vi "FreeCOM.vi"() -> ()   [LabVIEW 2014]
uses:
  <vilib>/Platform/TimedLoop/XDataNode/timing_clust.ctl
  <vilib>/Platform/TimedLoop/XDataNode/nitl_modes.ctl
  <vilib>/Platform/TimedLoop/XDataNode/wakeup.ctl
  <vilib>/Instr/_visa.llb/VISA Configure Serial Port (Instr).vi
  <vilib>/Utility/file.llb/Write To Spreadsheet File (string).vi
  <vilib>/Utility/file.llb/Write To Spreadsheet File (I64).vi
  <vilib>/Utility/file.llb/Read From Spreadsheet File (I64).vi
  <vilib>/Platform/TimedLoop/XDataNode/XDataNode.xnode
  <vilib>/Platform/TimedLoop/XDataNode/XDNodeRunTimeDep.lvlib
  <vilib>/Analysis/NI_AALBase.lvlib
  <vilib>/httpClient/LabVIEWHTTPClient.lvlib
  <vilib>/httpClient/POSTBuffer.vi
panel:
  out "字符串 2":string
  out "串口状态":bool
  out "百度纬度":dbl=50.0 format="%.10f"
  out "百度经度":dbl=50.0 format="%.10f"
  out "滤波后的历史数据":i16[][](array[numeric])
  out "04最新":i16[](array[numeric])
  out "基准时间":dbl format="%#_13g"
  out "存读的历史数据":i16[][](array[numeric])
  out "F2最新":i16[](array[numeric])
  out "F1最新":i16[](array[numeric])
  out "02最新":i16[](array[numeric])
  in  "选项卡控件":enum32{"采集界面", "地图", "设置"}(tab)
  out "波形图":i16[][](graph)
  in  "端口号":u16(ring) items=["COM1", "COM2", "COM3", "COM4", "COM5", "COM6", "COM7", "COM8", "COM9", "COM10"]
  in  "计时开关":bool
  in  "读取按钮":bool
  in  "保存按钮":bool
  out "转速":dbl(knob) scale=0.0..100.0
  out "轮速0":dbl(knob) scale=0.0..10.0
  out "档位":dbl format="%#_3g"
  out "水温":dbl(slide) scale=20.0..120.0
  out "电池电压":dbl(slide) scale=0.0..20.0
  out "节流阀位置":dbl(slide) scale=0.0..100.0
  out "前向加速度":dbl
  out "侧向加速度":dbl
  out "纵向加速度":dbl
  out "前向角速度":dbl
  out "侧向角速度":dbl
  out "纵向角速度":dbl
  out "误码":bool
  in  "open":bool
  in  "VISA资源名称":refnum<visa-resource-name>
  in  "波特率":u16(ring) caption="Baud" items=["115200", "9600"]
  out "时间差":dbl format="%#.3g秒"
  in  "侧向G值":cluster{dbl, dbl}(slide) caption="AccX图显" scale=-2.0..2.0
  in  "清除数据":bool
  in  "地图缩放":u8(slide) scale=1.0..19.0
  out "定位模式":string
  out "定位状态":dbl
  out "海拔":dbl
  in  "WebBrowser":refnum<k7>(container) caption="网页浏览器"
  out "纬度":dbl format="%#.10f"
  out "经度":dbl format="%#.10f"
  out "卫星数量":dbl
  out "地速":dbl
  out "航向":dbl
  out "航向图":picture caption="航向"
  in  "显示游标":bool
  in  "G值校准常量":dbl
  in  "串口模拟开关":bool
  out "FA数据接收（字符消息）":string caption="接收区"
  in  "发送区":string
  in  "send":bool
  in  "换行":bool
  out "TX":dbl
  out "RX":dbl
  in  "滤波系数调整":i16(slide) scale=0.0..5.0
  out "计数器":dbl
  out "历史数据05":i16[][](array[numeric])
  out "历史数据F2":i16[][](array[numeric])
  out "历史数据F1":i16[][](array[numeric])
  out "历史数据04":i16[][](array[numeric])
  out "历史数据03":i16[][](array[numeric])
  out "历史数据02":i16[][](array[numeric])
  out "历史数据01":i16[][](array[numeric])
  out "提取缓存":i64[](array[numeric])
  # "用户使用"
  # "Count"
  # "开发人员使用"
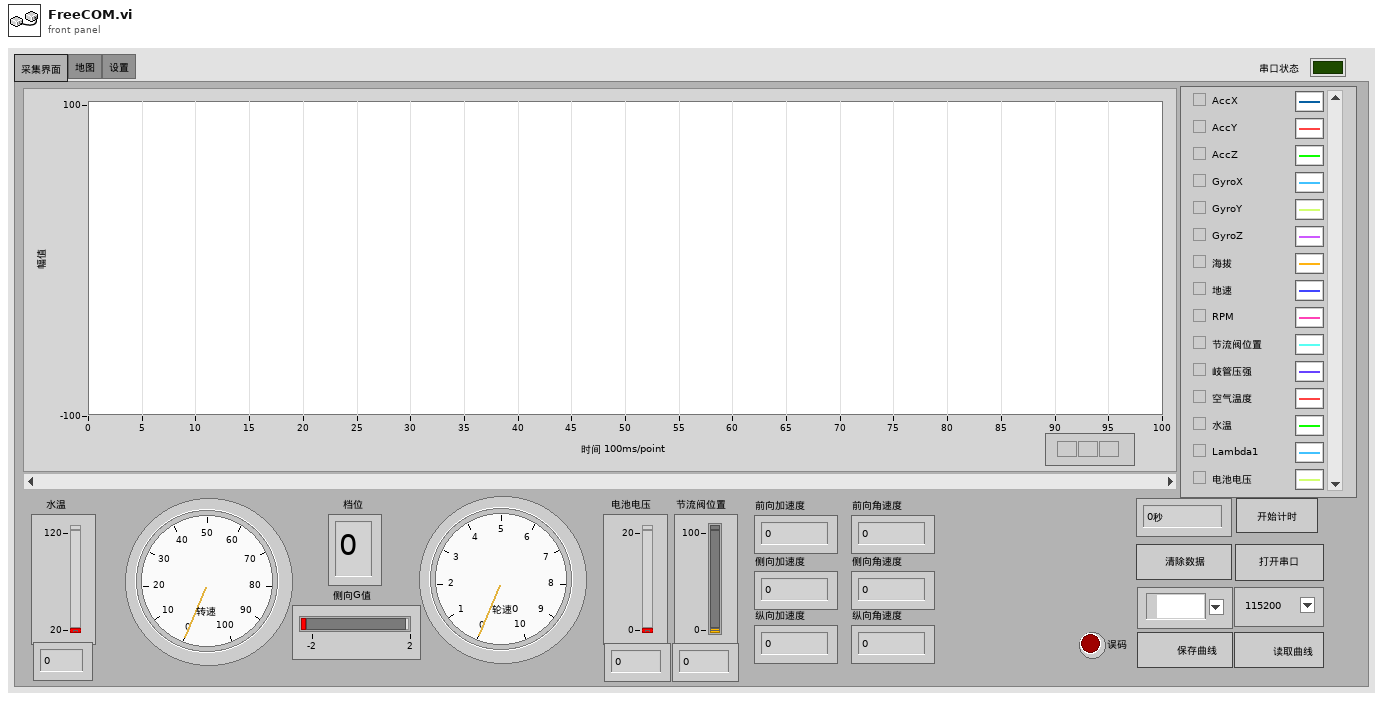
[diagram p1: front panel]
types:
  T1 = typedef "XDNodeRunTimeDep.lvlib/timing_clust.ctl" = cluster{"Expected End [f-1]":u64, "Actual End [f-1]":u64, "Finished Late? [f-1]":bool, "Expected End [i-1]":u64, "Actual End [i-1]":u64, "Finished Late? [i-1]":bool, "Expected Start [i]":u64, "Actual Start [i]":u64, "Expected Start [f]":u64, "Actual Start [f]":u64, "Source Name":string, "Structure Name":string, "Period":i64, "Deadline":i64, "Offset":i64, "Start":i64, "Priority":i32, "Timeout":i32, "Mode":T2, "Wakeup Reason":T3, "Error":errorcluster, "Source Type":string, "Secondary Source Type":string, "Global End Time":u64, "Global Start Time":u64, "Frame Duration":u64, "Iteration Duration":u64, "Assigned CPU":i32, "I/O Scan Engine Mode":u32}
  T2 = typedef "XDNodeRunTimeDep.lvlib/nitl_modes.ctl" = enum32{"No Change", "Process missed periods, maintain original phase", "Discard missed periods, maintain original phase", "Process missed periods, ignore original phase", "Discard missed periods, ignore original phase"}
  T3 = typedef "XDNodeRunTimeDep.lvlib/wakeup.ctl" = enum32{"Normal", "Aborted", "Asynchronous wakeup", "Timing source error", "Timed loop error", "Timeout"}
  T4 = cluster{"maximum":dbl, "minimum":dbl, "clip to min":bool, "log?(F)":bool, "grid color":u32, "plot color":u32, "format and precision":cluster{"format":enum8{"Decimal", "Scientific", "Engineering", "Binary", "Octal", "Hex"}, "precision":u8}, "visible section":u16}
  T5 = typedef "LabVIEWHTTPClient.lvlib/ClientHandle.ctl" = refnum<k1>
  T6 = typedef "LVBoundsTypeDef.ctl" = cluster{"Width":u32, "Height":u32}
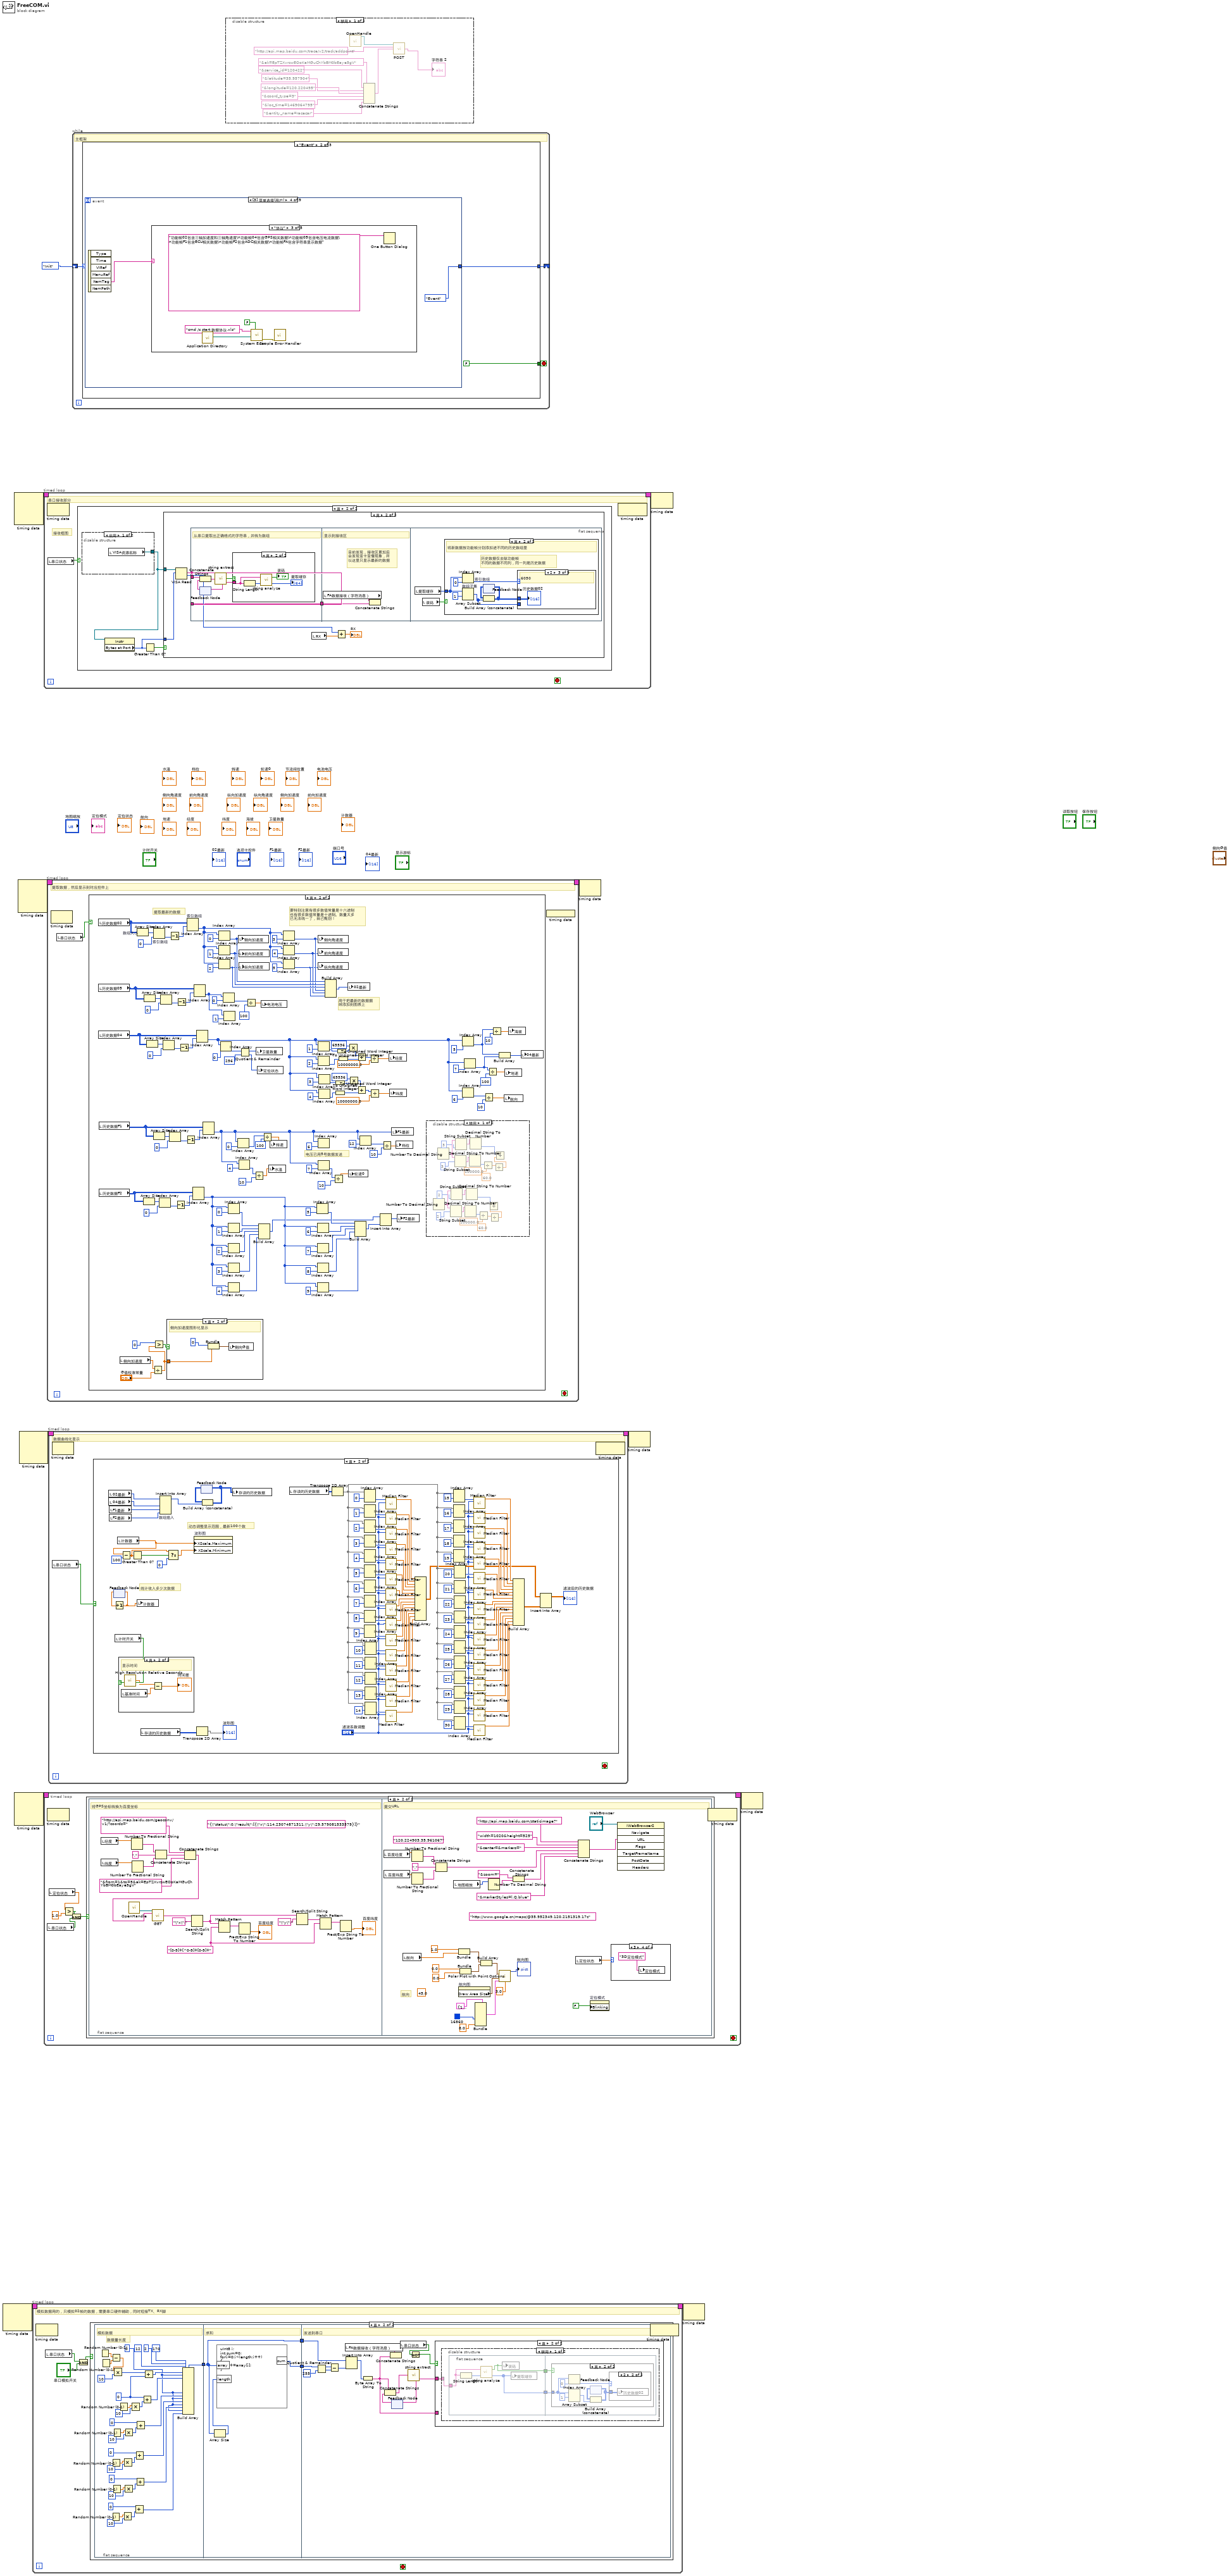
[diagram p0: block diagram]
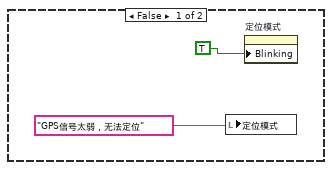
[diagram p3: hidden frame]
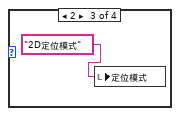
[diagram p6: hidden frame]
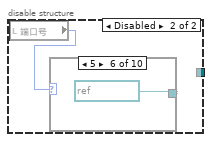
[diagram p10: hidden frame]
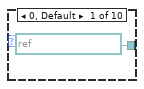
[diagram p11: hidden frame]
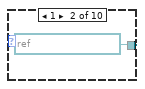
[diagram p12: hidden frame]
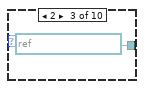
[diagram p13: hidden frame]
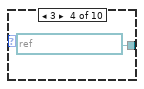
[diagram p14: hidden frame]
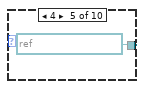
[diagram p15: hidden frame]
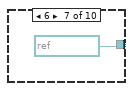
[diagram p16: hidden frame]
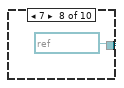
[diagram p17: hidden frame]
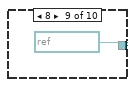
[diagram p18: hidden frame]
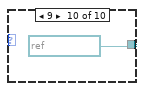
[diagram p19: hidden frame]
diagram:
  n1 = node-c288() -> (w8:T1)  [unwired: 3 in]
  n2 = node-c288() -> (w6:T1)  [unwired: 4 in]
  n3 = node-c288() -> (w2:T1)  [unwired: 4 in]
  n4 = node-c288() -> (w10:T1)  [unwired: 4 in]
  n5 = node-c288() -> (w4:T1)  [unwired: 4 in]
  n6 = timed-loop "定时循环" {
    timing: w8 -> [_]
    timing-out: [_] -> w7
    stop <- _ stop-if-true
    # "模拟数据用的，只模拟02帧的数据，需要串口硬件辅助，同时短接TX、RX脚"
    n7 = node-c288() -> ()  [unwired: 1 in, 1 out]
    n8 = local read "串口状态"() -> (w13:bool)
    n9 = And(x=w13, y="串口模拟开关") -> (x .and. y?=w12:bool)
    n10 = case shown="真" w12 {
      frame False {
      }
      frame True {
        n11 = flat-sequence "平铺式顺序结构" {
          tunnel: [w54] -> w19
          tunnel: w19 -> [w58]
          tunnel: [w57] -> w18
          tunnel: [w58] -> w17
          tunnel: w18 -> [w72]
          tunnel: w17 -> [w73]
          frame #0 {
            w46 = 0
            w24 = 0
            w55 = 170
            # "数据量长度"
            # "模拟数据"
            n12 = Random Number (0-1)() -> (number: 0 to 1=w22:dbl)
            n13 = Random Number (0-1)() -> (number: 0 to 1=w21:dbl)
            n14 = Random Number (0-1)() -> (number: 0 to 1=w28:dbl)
            n15 = Subtract(x=w22, y=w21) -> (x-y=w20:dbl)
            n16 = Random Number (0-1)() -> (number: 0 to 1=w38:dbl)
            n17 = Random Number (0-1)() -> (number: 0 to 1=w34:dbl)
            n18 = Random Number (0-1)() -> (number: 0 to 1=w43:dbl)
            n19 = Multiply ("乘")(x=w20, y=10) -> (x*y=w44:i16)
            n20 = Random Number (0-1)() -> (number: 0 to 1=w53:dbl)
            n21 = Multiply ("乘")(x=w28, y=10) -> (x*y=w26:u16)
            n22 = Multiply ("乘")(x=w38, y=10) -> (x*y=w36:u16)
            n23 = Multiply ("乘")(x=w34, y=10) -> (x*y=w32:u16)
            n24 = Multiply ("乘")(x=w43, y=10) -> (x*y=w41:u16)
            n25 = Multiply ("乘")(x=w53, y=10) -> (x*y=w51:u16)
            n26 = Add(x=0, y=w26) -> (x+y=w23:i32)
            n27 = Add(x=0, y=w36) -> (x+y=w30:i32)
            n28 = Add(x=0, y=w32) -> (x+y=w29:i32)
            n29 = Add(x=0, y=w41) -> (x+y=w39:i32)
            n30 = Add(x=w46, y=w51) -> (x+y=w50:i32)
            n31 = Add(x=w44, y=w46) -> (x+y=w45:i32)
            n32 = Build Array(w55, w55, 2, 12, w24, w45, w24, w50, w24, w39, w24, w30, w24, w29, w24, w23) -> (w54:i32[])
          }
          frame #1 {
            # "求和"
            n33 = Array Size(array=w58) -> (size(s)=w56:i32)
            n34 = formula code="uInt8 i;\nint sum=0;\nfor(i=0;i<length;i++)\n{\n sum+=array[i];\n}"("array"=w58, "length"=w56) -> ("sum"=w57:i32)
          }
          frame #2 {
            # "发送到串口"
            n35 = Quotient & Remainder(x=w72, y=255) -> (x-y*floor(x/y)=w70:i32, floor(x/y)=w69:i32)
            n36 = Subtract(x=w70, y=w69) -> (x-y=w68:i32)
            n37 = local read "FA数据接收（字符消息）"() -> (w63:string)
            n38 = Insert Into Array(array=w73, new element=w68) -> (w67:i32[])  [unwired: 1 in]
            n39 = Byte Array To String(unsigned byte array=w67) -> (string=w61:string)
            n40 = Concatenate Strings(w63, w61) -> ()  [unwired: 1 out]
            n41 = feedback #1() -> (w64:string)  [unwired: 1 in]
            n42 = Concatenate Strings(w61, w64) -> (w66:string)
            n43 = local read "串口状态"() -> (w60:bool)
            n44 = call "string extract.vi"("输入的串"=w66) -> ("输出的串"=w62:string, "剩余的串"=w65:string)  [unwired: 3 out]
            n45 = feedback-in #1(w65) -> ()
            n46 = Not(x=w60) -> (.not. x?=w59:bool)
            n47 = case shown="真" w59 {
              tunnel: w62 -> [_ w88]
              tunnel: w61 -> [w75 _]
              frame False {
                n48 = disable-structure shown="启用" {
                  disable-tunnel: [w76 _] -> w74
                  frame Enabled {
                    n49 = local read "VISA资源名称"() -> (w76:refnum<visa-resource-name>)
                  }
                  frame Disabled {
                    n50 = local read "端口号"() -> (w77:u16)
                    n51 = case shown="5" w77 {
                      tunnel: [refnum<visa-resource-name> "ASRL1::INSTR" ("VISA resource name") refnum<visa-resource-name> "ASRL2::INSTR" ("VISA resource name") refnum<visa-resource-name> "ASRL3::INSTR" ("VISA resource name") refnum<visa-resource-name> "ASRL4::INSTR" ("VISA resource name") refnum<visa-resource-name> "ASRL5::INSTR" ("VISA resource name") refnum<visa-resource-name> "COM6" ("VISA resource name") refnum<visa-resource-name> "COM7" ("VISA resource name") refnum<visa-resource-name> "COM8" ("VISA resource name") refnum<visa-resource-name> "COM9" ("VISA resource name") refnum<visa-resource-name> "COM10" ("VISA resource name")] -> _
                      frame 0, Default {
                      }
                      frame 1 {
                      }
                      frame 2 {
                      }
                      frame 3 {
                      }
                      frame 4 {
                      }
                      frame 5 {
                      }
                      frame 6 {
                      }
                      frame 7 {
                      }
                      frame 8 {
                      }
                      frame 9 {
                      }
                    }
                  }
                }
                n52 = VISA Write(VISA resource name=w74, write buffer=w75) -> ()  [unwired: 1 in, 3 out]
              }
              frame True {
                n53 = disable-structure shown="禁用" {
                  disable-tunnel: w88 -> [w89 _]
                  frame Disabled {
                    n54 = flat-sequence {
                      tunnel: w89 -> [w94]
                      tunnel: [w93] -> w91
                      tunnel: [w92] -> w90
                      tunnel: w91 -> [w97]
                      tunnel: w90 -> [w96]
                      frame #0 {
                        n55 = String Length(string=w94) -> (length=w95:i32)
                        n56 = call "string analyze.vi"("串的长度"=w95, "输入的串"=w94) -> ("输出的数组"=w92:i64[], "串正确"=w93:bool)
                        n57 = local write "误码"(w93) -> ()
                        n58 = local write "提取缓存"(w92) -> ()
                      }
                      frame #1 {
                        n59 = case shown="真" w97 {
                          tunnel: w96 -> [_ w100]
                          frame False {
                          }
                          frame True {
                            n60 = Index Array(array=w100, index=0) -> (element=w99:i64)
                            n61 = Array Subset(array=w100, index=1) -> (w104:i64[])  [unwired: 1 in]
                            n62 = feedback #2() -> (w101:i64[][])  [unwired: 1 in]
                            n63 = Build Array (concatenate)(w101, w104) -> (w98:i64[][])
                            n64 = feedback-in #2(w98) -> ()
                            n65 = case shown="2" w99 {
                              tunnel: w98 -> [_ w105]
                              frame 0, Default {
                              }
                              frame 2 {
                                n66 = local write "历史数据02"(w105) -> ()
                              }
                            }
                          }
                        }
                      }
                    }
                  }
                  frame Enabled {
                  }
                }
              }
            }
          }
        }
      }
    }
    n67 = node-c288() -> ()  [unwired: 1 in, 1 out]
  }
  n68 = timed-loop "定时循环" {
    timing: w6 -> [_]
    timing-out: [_] -> w5
    stop <- _ stop-if-true
    # "接收框图"
    # "串口接收部分"
    n69 = node-c288() -> ()  [unwired: 1 in, 1 out]
    n70 = local read "串口状态"() -> (w106:bool)
    n71 = case shown="真" w106 {
      frame False {
      }
      frame True {
        n72 = disable-structure shown="启用" {
          disable-tunnel: [w112 _] -> w109
          frame Enabled {
            n73 = local read "VISA资源名称"() -> (w112:refnum<visa-resource-name>)
          }
          frame Disabled {
            n74 = local read "端口号"() -> (w113:u16)
            n75 = case shown="5" w113 {
              tunnel: [refnum<visa-resource-name> "ASRL1::INSTR" ("VISA resource name") refnum<visa-resource-name> "ASRL2::INSTR" ("VISA resource name") refnum<visa-resource-name> "ASRL3::INSTR" ("VISA resource name") refnum<visa-resource-name> "ASRL4::INSTR" ("VISA resource name") refnum<visa-resource-name> "ASRL5::INSTR" ("VISA resource name") refnum<visa-resource-name> "COM6" ("VISA resource name") refnum<visa-resource-name> "COM7" ("VISA resource name") refnum<visa-resource-name> "COM8" ("VISA resource name") refnum<visa-resource-name> "COM9" ("VISA resource name") refnum<visa-resource-name> "COM10" ("VISA resource name")] -> _
              frame 0, Default {
              }
              frame 1 {
              }
              frame 2 {
              }
              frame 3 {
              }
              frame 4 {
              }
              frame 5 {
              }
              frame 6 {
              }
              frame 7 {
              }
              frame 8 {
              }
              frame 9 {
              }
            }
          }
        }
        n76 = property class="Instr"(reference=w109) -> ("Bytes at Port"=w111:u32)  [unwired: 1 in, 2 out]
        n77 = Greater Than 0?(x=w111) -> (x > 0?=w110:bool)
        n78 = case shown="真" w110 {
          tunnel: w109 -> [_ w130]
          tunnel: w111 -> [_ w127]
          frame False {
          }
          frame True {
            n79 = VISA Read(VISA resource name=w130, byte count=w127) -> (read buffer=w125:string, return count=w124:u32)  [unwired: 1 in, 2 out]
            n80 = flat-sequence "平铺式顺序结构" {
              tunnel: w125 -> [w132]
              tunnel: w125 -> [w131]
              tunnel: [w131] -> w126
              tunnel: w126 -> [w143]
              frame #0 {
                # "从串口提取出正确格式的字符串，并转为数组"
                n81 = feedback #3() -> (w133:string)  [unwired: 1 in]
                n82 = Concatenate Strings(w132, w133) -> (w134:string)
                n83 = call "string extract.vi"("输入的串"=w134) -> ("输出的串"=w137:string, "剩余的串"=w135:string, "输出的串非空"=w136:bool)  [unwired: 2 out]
                n84 = feedback-in #3(w135) -> ()
                n85 = case shown="真" w136 {
                  tunnel: w137 -> [_ w139]
                  frame False {
                    n86 = local write "误码"(FALSE) -> ()
                  }
                  frame True {
                    n87 = String Length(string=w139) -> (length=w142:i32)
                    n88 = call "string analyze.vi"("串的长度"=w142, "输入的串"=w139) -> ("输出的数组"=→"提取缓存":i64[], "串正确"=→"误码":bool)
                  }
                }
              }
              frame #1 {
                # "目前发现，接收区累加后\n会发现变卡变慢现象，所\n以这里只显示最新的数据"
                # "显示到接收区"
                n89 = local read "FA数据接收（字符消息）"() -> (w144:string)
                n90 = Concatenate Strings(w144, w143) -> ()  [unwired: 1 out]
              }
              frame #2 {
                n91 = local read "提取缓存"() -> (w146:i64[])
                n92 = local read "误码"() -> (w145:bool)
                n93 = case "条件结构" shown="真" w145 {
                  tunnel: w146 -> [_ w150]
                  frame False {
                  }
                  frame True {
                    # "历史数据仅去除功能帧\n不同的数据不同列，同一列是历史数据"
                    # "将新数据按功能帧分别添加进不同的历史数组里"
                    n94 = Index Array "索引数组"(array=w150, index=0) -> (element=w149:i64)
                    n95 = Array Subset "数组子集"(array=w150, index=1) -> (w147:i64[])  [unwired: 1 in]
                    n96 = feedback #4() -> (w153:i64[][])  [unwired: 1 in]
                    n97 = Build Array (concatenate)(w153, w147) -> (w148:i64[][])
                    n98 = feedback-in #4(w148) -> ()
                    n99 = case "条件结构" shown="2" w149 {
                      tunnel: w148 -> [_ w154 w155 w156 w157 w158 w159 w160 _]
                      tunnel: w147 -> [_ _ _ _ _ _ _ _ w161]
                      frame 0, Default {
                      }
                      frame 1 {
                        # "ATT"
                        "历史数据01" <- w154
                      }
                      frame 2 {
                        # "6050"
                        "历史数据02" <- w155
                      }
                      frame 3 {
                        "历史数据03" <- w156
                      }
                      frame 4 {
                        # "GPS"
                        "历史数据04" <- w157
                      }
                      frame 5 {
                        "历史数据05" <- w158
                      }
                      frame 241 {
                        # "Motec"
                        "历史数据F1" <- w159
                      }
                      frame 242 {
                        # "ADC"
                        "历史数据F2" <- w160
                      }
                      frame 250 {
                        # "FA的数据转为字符"
                        n100 = Byte Array To String(unsigned byte array=w161) -> (string=→"FA数据接收（字符消息）":string)
                      }
                    }
                  }
                }
              }
            }
            n101 = local read "RX"() -> (w129:dbl)
            n102 = Add(x=w124, y=w129) -> (x+y=→"RX":dbl)
          }
        }
      }
    }
    n103 = node-c288() -> ()  [unwired: 1 in, 1 out]
  }
  n104 = timed-loop {
    timing: w2 -> [_]
    timing-out: [_] -> w1
    stop <- _ stop-if-true
    n105 = node-c288() -> ()  [unwired: 1 in, 1 out]
    n106 = local read "串口状态"() -> (w164:bool)
    n107 = local read "定位状态"() -> (w167:dbl)
    n108 = Greater?(x=w167, y=1.0) -> (0:w165:bool)
    n109 = And(x=w165, y=w164) -> (x .and. y?=w163:bool)
    n110 = case shown="真" w163 {
      frame False {
        n111 = local write "定位模式"("GPS信号太弱，无法定位") -> ()
        n112 = property on="定位模式" class="Str"("Blinking"=TRUE) -> ()  [unwired: 2 in, 2 out]
      }
      frame True {
        n113 = flat-sequence "平铺式顺序结构" {
          frame #0 {
            w189 = "[0-9]+[^0-9]+[0-9]+"
            (unwired) "{\"status\":0,\"result\":[{\"x\":114.23074871311,\"y\":29.579081533579}]}" ("字符串 2")
            # "将GPS坐标转换为百度坐标"
            n114 = local read "经度"() -> (w174:dbl)
            n115 = local read "纬度"() -> (w175:dbl)
            n116 = call <vilib>:"OpenHandle.vi"() -> ("client handle out"=w187:T5)  [unwired: 14 in, 1 out]
            n117 = Number To Fractional String(number=w174) -> (F-format string=w178:string)  [unwired: 3 in]
            n118 = Number To Fractional String(number=w175) -> (F-format string=w176:string)  [unwired: 3 in]
            n119 = Concatenate Strings(w178, ",", w176) -> (w172:string)
            n120 = Concatenate Strings("http://api.map.baidu.com/geoconv/v1/?coords=", w172, "&from=1&to=5&ak=EpTZXvrzwEOoKaMGuChYbBM0bEaye5gV") -> (w170:string)
            n121 = call <vilib>:"GET.vi"("client handle"=w187, "url"=w170) -> ("body"=w188:string)  [unwired: 10 in, 3 out]
            n122 = Search/Split String(string=w188, search string/char (-)="\"x\":") -> (match + rest of string=w185:string)  [unwired: 1 in, 2 out]
            n123 = Match Pattern(string=w185, regular expression=w189) -> (match substring=w186:string)  [unwired: 1 in, 3 out]
            n124 = Fract/Exp String To Number(string=w186) -> (number=→"百度经度":dbl)  [unwired: 3 in, 1 out]
            n125 = Search/Split String(string=w185, search string/char (-)="\"y\":") -> (match + rest of string=w182:string)  [unwired: 1 in, 2 out]
            n126 = Match Pattern(string=w182, regular expression=w189) -> (match substring=w184:string)  [unwired: 1 in, 3 out]
            n127 = Fract/Exp String To Number(string=w184) -> (number=→"百度纬度":dbl)  [unwired: 3 in, 1 out]
          }
          frame #1 {
            (unwired) "http://www.google.cn/maps/@35.952349,120.2151319,17z"
            (unwired) 45.0
            (unwired) "120.224903,35.961067"
            # "航向"
            # "提交URL"
            n128 = local read "百度经度"() -> (w202:dbl)
            n129 = local read "百度纬度"() -> (w201:dbl)
            n130 = local read "航向"() -> (w191:dbl)
            n131 = Number To Fractional String(number=w202) -> (F-format string=w200:string)  [unwired: 3 in]
            n132 = Number To Fractional String(number=w201) -> (F-format string=w198:string)  [unwired: 3 in]
            n133 = Concatenate Strings(w200, ",", w198) -> (w192:string)
            n134 = local read "地图缩放"() -> (w196:u8)
            n135 = Bundle(1.0, "航向"=w191) -> (w209:cluster{dbl, " 航向":dbl})  [unwired: 1 in]
            n136 = property on="航向图" class="Pict"() -> ("Draw Area Size"=w205:T6)  [unwired: 2 in, 2 out]
            n137 = Bundle(0.0, 0.0) -> (w210:cluster{dbl, dbl})  [unwired: 1 in]
            n138 = Bundle(cluster=T4 {"maximum"=1.0, "minimum"=0.0, "clip to min"=FALSE, "log?(F)"=FALSE, "grid color"=6710886, "plot color"=65280, "format and precision"={"format"=enum."Decimal", "precision"=1}, "visible section"=0} ("Polar Graph Attributes"), "plot color"=u32 16860, "visible section"=8.0) -> (w213:T4)  [unwired: 6 in]
            n139 = Build Array(w209, w210) -> (w211:cluster{dbl, " 航向":dbl}[])
            n140 = Number To Decimal String(number=w196) -> (decimal integer string=w195:string)  [unwired: 1 in]
            n141 = call <vilib>:"Polar Plot with Point Options.vi"("data array [mag, phase (deg)]"=w211, "dimensions (w,h)"=w205, "polar attributes"=w213, "Size"=3.0) -> ("new picture"=→"航向图":picture)  [unwired: 11 in]
            n142 = Concatenate Strings("&zoom=", w195) -> (w194:string)
            n143 = local read "定位状态"() -> (w203:dbl)
            n144 = Concatenate Strings("http://api.map.baidu.com/staticimage?", "width=1020&height=525", "&center=&markers=", w192, w194, "&markerStyles=l,Q,blue") -> (w190:string)
            n145 = property on="定位模式" class="Str"("Blinking"=FALSE) -> ()  [unwired: 2 in, 2 out]
            n146 = case shown="3" w203 {
              frame 0, Default {
              }
              frame 1 {
              }
              frame 2 {
                n147 = local write "定位模式"("2D定位模式") -> ()
              }
              frame 3 {
                n148 = local write "定位模式"("3D定位模式") -> ()
              }
            }
            n149 = invoke class="IWebBrowser2" method="Navigate"(reference="WebBrowser", "URL"=w190) -> ()  [unwired: 6 in, 8 out]
          }
        }
      }
    }
    n150 = node-c288() -> ()  [unwired: 1 in, 1 out]
  }
  n151 = timed-loop "定时循环" {
    timing: w10 -> [_]
    timing-out: [_] -> w9
    stop <- _ stop-if-true
    # "提取数据，然后显示到对应控件上"
    n152 = node-c288() -> ()  [unwired: 1 in, 1 out]
    n153 = local read "串口状态"() -> (w226:bool)
    n154 = case shown="真" w226 {
      frame False {
      }
      frame True {
        # "要特别注意有很多数值常量是十六进制\n也有很多数值常量是十进制。数量太多\n已无法统一了，自己甄别！"
        # "用于把最新的数据捆\n绑添加到图表上"
        # "提取最新的数据"
        # "电压已用5号数据发送"
        n155 = local read "历史数据02"() -> (w299:i16[][])
        n156 = local read "历史数据05"() -> (w357:i16[][])
        n157 = local read "历史数据04"() -> (w318:i16[][])
        n158 = local read "历史数据F1"() -> (w356:i16[][])
        n159 = local read "历史数据F2"() -> (w345:i16[][])
        n160 = local read "侧向加速度"() -> (w275:dbl)
        n161 = Array Size "数组大小"(array=w299) -> (size(s)=w298:i32[])
        n162 = Array Size(array=w345) -> (size(s)=w341:i32[])
        n163 = Array Size(array=w357) -> (size(s)=w309:i32[])
        n164 = Array Size(array=w318) -> (size(s)=w314:i32[])
        n165 = Divide(x=w275, y="G值校准常量") -> (x/y=w274:dbl)
        n166 = Index Array "索引数组"(array=w298, index=0) -> (element=w301:i32)
        n167 = Array Size(array=w356) -> (size(s)=w332:i32[])
        n168 = Greater?(x=i16 0, y=w274) -> (0:w282:bool)
        n169 = Index Array(array=w341, index=0) -> (element=w343:i32)
        n170 = Index Array(array=w309, index=0) -> (element=w311:i32)
        n171 = Index Array(array=w314, index=0) -> (element=w316:i32)
        n172 = case "条件结构" shown="真" w282 {
          tunnel: w274 -> [w381 w384]
          frame False {
            n173 = Bundle(w381, i16 0) -> (w382:cluster{dbl, i16})  [unwired: 1 in]
            n174 = local write "侧向G值"(w382) -> ()
          }
          frame True {
            # "侧向加速度图形化显示"
            n175 = Bundle(i16 0, w384) -> (w385:cluster{i16, dbl})  [unwired: 1 in]
            n176 = local write "侧向G值"(w385) -> ()
          }
        }
        n177 = Decrement(x=w301) -> (x-1=w302:i32)
        n178 = Index Array(array=w332, index=0) -> (element=w334:i32)
        n179 = Decrement(x=w343) -> (x-1=w344:i32)
        n180 = Decrement(x=w311) -> (x-1=w312:i32)
        n181 = Decrement(x=w316) -> (x-1=w317:i32)
        n182 = Decrement(x=w334) -> (x-1=w335:i32)
        n183 = Index Array "索引数组"(array=w299, index (row)=w302) -> (element=w283:i16[])  [unwired: 1 in]
        n184 = Index Array(array=w345, index (row)=w344) -> (element=w359:i16[])  [unwired: 1 in]
        n185 = Index Array(array=w357, index (row)=w312) -> (element=w297:i16[])  [unwired: 1 in]
        n186 = Index Array(array=w318, index (row)=w317) -> (element=w243:i16[])  [unwired: 1 in]
        n187 = Index Array(array=w356, index (row)=w335) -> (element=w264:i16[])  [unwired: 1 in]
        n188 = Index Array(array=w283, index=0) -> (element=w272:i16)
        n189 = Index Array(array=w283, index=1) -> (element=w271:i16)
        n190 = Index Array(array=w283, index=2) -> (element=w270:i16)
        n191 = Index Array(array=w243, index=0) -> (element=w321:i16)
        n192 = Index Array(array=w297, index=0) -> (element=w262:i16)
        n193 = Index Array(array=w297, index=1) -> ()  [unwired: 1 out]
        n194 = Index Array(array=w359, index=0) -> (element=w296:i16)
        n195 = Index Array(array=w359, index=1) -> (element=w295:i16)
        n196 = Index Array(array=w359, index=2) -> (element=w293:i16)
        n197 = Index Array(array=w359, index=3) -> (element=w294:i16)
        n198 = Index Array(array=w359, index=4) -> (element=w292:i16)
        n199 = Index Array(array=w264, index=0) -> (element=w280:i16)
        n200 = local write "侧向加速度"(w272) -> ()
        n201 = local write "前向加速度"(w271) -> ()
        n202 = local write "纵向加速度"(w270) -> ()
        n203 = Index Array(array=w264, index=4) -> (element=w259:i16)
        n204 = Quotient & Remainder(x=w321, y=256) -> (x-y*floor(x/y)=w322:i32, floor(x/y)=w241:i32)
        n205 = Divide(x=w262, y=100) -> (x/y=w260:dbl)
        n206 = Divide(x=w259, y=10) -> (x/y=w257:dbl)
        n207 = local write "卫星数量"(w322) -> ()
        n208 = local write "定位状态"(w241) -> ()
        n209 = Build Array(w296, w295, w293, w294, w292) -> (w286:i16[])
        n210 = local write "电池电压"(w260) -> ()
        n211 = Divide(x=w280, y=100) -> (x/y=w278:dbl)
        n212 = local write "水温"(w257) -> ()
        n213 = local write "转速"(w278) -> ()
        n214 = Index Array(array=w283, index=3) -> (element=w269:i16)
        n215 = Index Array(array=w283, index=4) -> (element=w268:i16)
        n216 = Index Array(array=w283, index=5) -> (element=w267:i16)
        n217 = Index Array(array=w359, index=5) -> (element=w291:i16)
        n218 = Index Array(array=w359, index=6) -> (element=w290:i16)
        n219 = Index Array(array=w359, index=7) -> (element=w289:i16)
        n220 = Index Array(array=w359, index=8) -> (element=w288:i16)
        n221 = Index Array(array=w359, index=9) -> (element=w287:i16)
        n222 = local write "侧向角速度"(w269) -> ()
        n223 = local write "前向角速度"(w268) -> ()
        n224 = local write "纵向角速度"(w267) -> ()
        n225 = Index Array(array=w243, index=1) -> (element=w232:i16)
        n226 = Index Array(array=w243, index=2) -> (element=w234:i16)
        n227 = Index Array(array=w264, index=6) -> ()  [unwired: 1 out]
        n228 = Index Array(array=w264, index=7) -> (element=w255:i16)
        n229 = Index Array(array=w243, index=3) -> (element=w230:i16)
        n230 = Index Array(array=w243, index=4) -> (element=w228:i16)
        n231 = Build Array(w272, w271, w270, w269, w268, w267) -> (w266:i16[])
        n232 = Divide(x=w255, y=10) -> (x/y=w254:dbl)
        n233 = To Unsigned Word Integer(number=w230) -> (unsigned 16bit integer=w229:u16)
        n234 = To Unsigned Word Integer(number=w228) -> (unsigned 16bit integer=w227:u16)
        n235 = To Unsigned Word Integer(number=w232) -> (unsigned 16bit integer=w231:u16)
        n236 = To Unsigned Word Integer(number=w234) -> (unsigned 16bit integer=w233:u16)
        n237 = local write "02最新"(w266) -> ()
        n238 = Multiply(x=65536, y=w231) -> (x*y=w253:i32)
        n239 = Multiply(x=65536, y=w229) -> (x*y=w329:i32)
        n240 = local write "轮速0"(w254) -> ()
        n241 = Build Array(w291, w290, w289, w288, w287) -> (w285:i16[])
        n242 = Add(x=w253, y=w233) -> (x+y=w240:i32)
        n243 = Add(x=w329, y=w227) -> (x+y=w237:i32)
        n244 = Index Array(array=w264, index=12) -> (element=w273:i16)
        n245 = Divide(x=w240, y=10000000.0) -> (x/y=w238:dbl)
        n246 = Divide(x=w237, y=10000000.0) -> (x/y=w235:dbl)
        n247 = Insert Into Array(array=w286, new element=w285) -> (w284:i16[])  [unwired: 1 in]
        n248 = Divide(x=w273, y=10) -> (x/y=w276:dbl)
        n249 = local write "经度"(w238) -> ()
        n250 = local write "纬度"(w235) -> ()
        n251 = local write "F1最新"(w264) -> ()
        n252 = local write "档位"(w276) -> ()
        n253 = local write "F2最新"(w284) -> ()
        n254 = disable-structure shown="禁用" {
          frame Disabled {
            (unwired) 60.0
            (unwired) 60.0
            n255 = Number To Decimal String() -> (decimal integer string=w365:string)  [unwired: 2 in]
            n256 = Number To Decimal String() -> (decimal integer string=w375:string)  [unwired: 2 in]
            n257 = String Subset(string=w365, offset (0)=2) -> (substring=w369:string)  [unwired: 1 in]
            n258 = String Subset(string=w365, length (rest)=2) -> (substring=w364:string)  [unwired: 1 in]
            n259 = String Subset(string=w375, offset (0)=3) -> (substring=w379:string)  [unwired: 1 in]
            n260 = String Subset(string=w375, length (rest)=3) -> (substring=w374:string)  [unwired: 1 in]
            n261 = Decimal String To Number(string=w369) -> (number=w368:i32)  [unwired: 2 in, 1 out]
            n262 = Decimal String To Number(string=w364) -> (number=w361:i32)  [unwired: 2 in, 1 out]
            n263 = Decimal String To Number(string=w379) -> (number=w378:i32)  [unwired: 2 in, 1 out]
            n264 = Decimal String To Number(string=w374) -> (number=w371:i32)  [unwired: 2 in, 1 out]
            n265 = Divide(x=w368, y=100000.0) -> (x/y=w366:dbl)
            n266 = Divide(x=w378, y=100000.0) -> (x/y=w376:dbl)
            n267 = Divide(x=w366) -> (x/y=w362:dbl)  [unwired: 1 in]
            n268 = Add(x=w361, y=w362) -> (x+y=w360:dbl)
            n269 = Divide(x=w376) -> (x/y=w372:dbl)  [unwired: 1 in]
            n270 = Add(x=w371, y=w372) -> ()  [unwired: 1 out]
          }
          frame Enabled {
          }
        }
        n271 = Index Array(array=w243, index=6) -> (element=w245:i16)
        n272 = Index Array(array=w243, index=5) -> (element=w252:i16)
        n273 = Index Array(array=w243, index=7) -> (element=w248:i16)
        n274 = Divide(x=w245, y=10) -> (x/y=w242:dbl)
        n275 = Divide(x=w248, y=100) -> (x/y=w247:dbl)
        n276 = Divide(x=w252, y=10) -> (x/y=w250:dbl)
        n277 = Build Array(w252, w248) -> (w265:i16[])
        n278 = local write "航向"(w242) -> ()
        n279 = local write "地速"(w247) -> ()
        n280 = local write "海拔"(w250) -> ()
        n281 = local write "04最新"(w265) -> ()
      }
    }
    n282 = node-c288() -> ()  [unwired: 1 out]
  }
  n283 = timed-loop "定时循环" {
    timing: w4 -> [_]
    timing-out: [_] -> w3
    stop <- _ stop-if-true
    # "数据曲线化显示"
    n284 = node-c288() -> ()  [unwired: 1 in, 1 out]
    n285 = local read "串口状态"() -> (w389:bool)
    n286 = case shown="真" w389 {
      frame False {
      }
      frame True {
        # "动态调整显示范围，最新100个数"
        # "统计收入多少次数据"
        n287 = local read "02最新"() -> (w503:i16[])
        n288 = local read "04最新"() -> (w502:i16[])
        n289 = local read "F1最新"() -> (w501:i16[])
        n290 = local read "F2最新"() -> (w500:i16[])
        n291 = feedback #5() -> (w493:dbl)  [unwired: 1 in]
        n292 = Increment(x=w493) -> (x+1=w492:dbl)
        n293 = feedback-in #5(w492) -> ()
        n294 = local read "计时开关"() -> (w491:bool)
        n295 = local read "计数器"() -> (w499:dbl)
        n296 = case "条件结构" shown="真" w491 {
          frame False {
          }
          frame True {
            # "显示时间"
            n297 = local read "基准时间"() -> (w509:dbl)
            n298 = call <vilib>:"High Resolution Relative Seconds.vi"() -> ("relative seconds"=w508:dbl)
            n299 = Subtract(x=w508, y=w509) -> (x-y=→"时间差":dbl)
          }
        }
        n300 = Subtract(x=w499, y=i16 100) -> (x-y=w494:dbl)
        n301 = Greater Than 0?(x=w494) -> (x > 0?=w497:bool)
        n302 = local write "计数器"(w492) -> ()
        n303 = local read "存读的历史数据"() -> (w490:i16[][])
        n304 = Insert Into Array "数组插入"(array=w503, new element #1=w502, new element #2=w501, new element #3=w500) -> (w505:i16[])  [unwired: 1 in]
        n305 = Select(t=w494, s=w497, f=i16 0) -> (s? t:f=w496:dbl)
        n306 = property on="波形图" class="WFGraph (严格)"("XScale.Maximum"=w499, "XScale.Minimum"=w496) -> ()  [unwired: 2 in, 2 out]
        n307 = Transpose 2D Array(2D array=w490) -> (transposed array=→"波形图":i16[][])
        n308 = feedback #6() -> (w504:i16[][])  [unwired: 1 in]
        n309 = Build Array (concatenate)(w504, w505) -> (w506:i16[][])
        n310 = feedback-in #6(w506) -> ()
        n311 = local write "存读的历史数据"(w506) -> ()
        n312 = local read "存读的历史数据"() -> (w488:i16[][])
        n313 = Transpose 2D Array(2D array=w488) -> (transposed array=w441:i16[][])
        n314 = Index Array(array=w441, index (row)=i16 0) -> (element=w456:i16[])  [unwired: 1 in]
        n315 = Index Array(array=w441, index (row)=i16 1) -> (element=w454:i16[])  [unwired: 1 in]
        n316 = Index Array(array=w441, index (row)=i16 2) -> (element=w453:i16[])  [unwired: 1 in]
        n317 = Index Array(array=w441, index (row)=i16 3) -> (element=w452:i16[])  [unwired: 1 in]
        n318 = Index Array(array=w441, index (row)=i16 4) -> (element=w451:i16[])  [unwired: 1 in]
        n319 = Index Array(array=w441, index (row)=i16 5) -> (element=w450:i16[])  [unwired: 1 in]
        n320 = Index Array(array=w441, index (row)=i16 6) -> (element=w449:i16[])  [unwired: 1 in]
        n321 = Index Array(array=w441, index (row)=i16 7) -> (element=w448:i16[])  [unwired: 1 in]
        n322 = Index Array(array=w441, index (row)=i16 8) -> (element=w447:i16[])  [unwired: 1 in]
        n323 = Index Array(array=w441, index (row)=i16 9) -> (element=w446:i16[])  [unwired: 1 in]
        n324 = Index Array(array=w441, index (row)=i16 10) -> (element=w445:i16[])  [unwired: 1 in]
        n325 = Index Array(array=w441, index (row)=i16 11) -> (element=w444:i16[])  [unwired: 1 in]
        n326 = Index Array(array=w441, index (row)=i16 12) -> (element=w443:i16[])  [unwired: 1 in]
        n327 = Index Array(array=w441, index (row)=i16 13) -> (element=w442:i16[])  [unwired: 1 in]
        n328 = Index Array(array=w441, index (row)=i16 14) -> (element=w455:i16[])  [unwired: 1 in]
        n329 = call <vilib>:"Median Filter.vi"("left rank"="滤波系数调整", "X"=w456) -> ("Filtered X"=w424:dbl[])  [unwired: 8 in, 1 out]
        n330 = call <vilib>:"Median Filter.vi"("left rank"="滤波系数调整", "X"=w454) -> ("Filtered X"=w423:dbl[])  [unwired: 8 in, 1 out]
        n331 = call <vilib>:"Median Filter.vi"("left rank"="滤波系数调整", "X"=w453) -> ("Filtered X"=w422:dbl[])  [unwired: 8 in, 1 out]
        n332 = call <vilib>:"Median Filter.vi"("left rank"="滤波系数调整", "X"=w452) -> ("Filtered X"=w421:dbl[])  [unwired: 8 in, 1 out]
        n333 = call <vilib>:"Median Filter.vi"("left rank"="滤波系数调整", "X"=w451) -> ("Filtered X"=w420:dbl[])  [unwired: 8 in, 1 out]
        n334 = call <vilib>:"Median Filter.vi"("left rank"="滤波系数调整", "X"=w450) -> ("Filtered X"=w419:dbl[])  [unwired: 8 in, 1 out]
        n335 = call <vilib>:"Median Filter.vi"("left rank"="滤波系数调整", "X"=w449) -> ("Filtered X"=w418:dbl[])  [unwired: 8 in, 1 out]
        n336 = call <vilib>:"Median Filter.vi"("left rank"="滤波系数调整", "X"=w448) -> ("Filtered X"=w417:dbl[])  [unwired: 8 in, 1 out]
        n337 = call <vilib>:"Median Filter.vi"("left rank"="滤波系数调整", "X"=w447) -> ("Filtered X"=w416:dbl[])  [unwired: 8 in, 1 out]
        n338 = call <vilib>:"Median Filter.vi"("left rank"="滤波系数调整", "X"=w446) -> ("Filtered X"=w415:dbl[])  [unwired: 8 in, 1 out]
        n339 = call <vilib>:"Median Filter.vi"("left rank"="滤波系数调整", "X"=w445) -> ("Filtered X"=w414:dbl[])  [unwired: 8 in, 1 out]
        n340 = call <vilib>:"Median Filter.vi"("left rank"="滤波系数调整", "X"=w444) -> ("Filtered X"=w413:dbl[])  [unwired: 8 in, 1 out]
        n341 = call <vilib>:"Median Filter.vi"("left rank"="滤波系数调整", "X"=w443) -> ("Filtered X"=w412:dbl[])  [unwired: 8 in, 1 out]
        n342 = call <vilib>:"Median Filter.vi"("left rank"="滤波系数调整", "X"=w442) -> ("Filtered X"=w411:dbl[])  [unwired: 8 in, 1 out]
        n343 = call <vilib>:"Median Filter.vi"("left rank"="滤波系数调整", "X"=w455) -> ("Filtered X"=w410:dbl[])  [unwired: 8 in, 1 out]
        n344 = Build Array(w424, w423, w422, w421, w420, w419, w418, w417, w416, w415, w414, w413, w412, w411, w410) -> (w393:dbl[][])
        n345 = Index Array(array=w441, index (row)=i16 15) -> (element=w440:i16[])  [unwired: 1 in]
        n346 = Index Array(array=w441, index (row)=i16 16) -> (element=w439:i16[])  [unwired: 1 in]
        n347 = Index Array(array=w441, index (row)=i16 17) -> (element=w438:i16[])  [unwired: 1 in]
        n348 = Index Array(array=w441, index (row)=i16 18) -> (element=w437:i16[])  [unwired: 1 in]
        n349 = Index Array(array=w441, index (row)=i16 19) -> (element=w436:i16[])  [unwired: 1 in]
        n350 = Index Array(array=w441, index (row)=i16 20) -> (element=w435:i16[])  [unwired: 1 in]
        n351 = Index Array(array=w441, index (row)=i16 21) -> (element=w434:i16[])  [unwired: 1 in]
        n352 = Index Array(array=w441, index (row)=i16 22) -> (element=w433:i16[])  [unwired: 1 in]
        n353 = Index Array(array=w441, index (row)=i16 23) -> (element=w432:i16[])  [unwired: 1 in]
        n354 = Index Array(array=w441, index (row)=i16 24) -> (element=w431:i16[])  [unwired: 1 in]
        n355 = Index Array(array=w441, index (row)=i16 25) -> (element=w430:i16[])  [unwired: 1 in]
        n356 = Index Array(array=w441, index (row)=i16 26) -> (element=w429:i16[])  [unwired: 1 in]
        n357 = Index Array(array=w441, index (row)=i16 27) -> (element=w428:i16[])  [unwired: 1 in]
        n358 = Index Array(array=w441, index (row)=i16 28) -> (element=w427:i16[])  [unwired: 1 in]
        n359 = Index Array(array=w441, index (row)=i16 29) -> (element=w426:i16[])  [unwired: 1 in]
        n360 = Index Array(array=w441, index (row)=i16 30) -> (element=w425:i16[])  [unwired: 1 in]
        n361 = call <vilib>:"Median Filter.vi"("left rank"="滤波系数调整", "X"=w440) -> ("Filtered X"=w409:dbl[])  [unwired: 8 in, 1 out]
        n362 = call <vilib>:"Median Filter.vi"("left rank"="滤波系数调整", "X"=w439) -> ("Filtered X"=w408:dbl[])  [unwired: 8 in, 1 out]
        n363 = call <vilib>:"Median Filter.vi"("left rank"="滤波系数调整", "X"=w438) -> ("Filtered X"=w407:dbl[])  [unwired: 8 in, 1 out]
        n364 = call <vilib>:"Median Filter.vi"("left rank"="滤波系数调整", "X"=w437) -> ("Filtered X"=w406:dbl[])  [unwired: 8 in, 1 out]
        n365 = call <vilib>:"Median Filter.vi"("left rank"="滤波系数调整", "X"=w436) -> ("Filtered X"=w405:dbl[])  [unwired: 8 in, 1 out]
        n366 = call <vilib>:"Median Filter.vi"("left rank"="滤波系数调整", "X"=w435) -> ("Filtered X"=w404:dbl[])  [unwired: 8 in, 1 out]
        n367 = call <vilib>:"Median Filter.vi"("left rank"="滤波系数调整", "X"=w434) -> ("Filtered X"=w403:dbl[])  [unwired: 8 in, 1 out]
        n368 = call <vilib>:"Median Filter.vi"("left rank"="滤波系数调整", "X"=w433) -> ("Filtered X"=w402:dbl[])  [unwired: 8 in, 1 out]
        n369 = call <vilib>:"Median Filter.vi"("left rank"="滤波系数调整", "X"=w432) -> ("Filtered X"=w401:dbl[])  [unwired: 8 in, 1 out]
        n370 = call <vilib>:"Median Filter.vi"("left rank"="滤波系数调整", "X"=w431) -> ("Filtered X"=w400:dbl[])  [unwired: 8 in, 1 out]
        n371 = call <vilib>:"Median Filter.vi"("left rank"="滤波系数调整", "X"=w430) -> ("Filtered X"=w399:dbl[])  [unwired: 8 in, 1 out]
        n372 = call <vilib>:"Median Filter.vi"("left rank"="滤波系数调整", "X"=w429) -> ("Filtered X"=w398:dbl[])  [unwired: 8 in, 1 out]
        n373 = call <vilib>:"Median Filter.vi"("left rank"="滤波系数调整", "X"=w428) -> ("Filtered X"=w397:dbl[])  [unwired: 8 in, 1 out]
        n374 = call <vilib>:"Median Filter.vi"("left rank"="滤波系数调整", "X"=w427) -> ("Filtered X"=w396:dbl[])  [unwired: 8 in, 1 out]
        n375 = call <vilib>:"Median Filter.vi"("left rank"="滤波系数调整", "X"=w426) -> ("Filtered X"=w395:dbl[])  [unwired: 8 in, 1 out]
        n376 = call <vilib>:"Median Filter.vi"("left rank"="滤波系数调整", "X"=w425) -> ("Filtered X"=w394:dbl[])  [unwired: 8 in, 1 out]
        n377 = Build Array(w409, w408, w407, w406, w405, w404, w403, w402, w401, w400, w399, w398, w397, w396, w395, w394) -> (w392:dbl[][])
        n378 = Insert Into Array(array=w393, new element=w392) -> (→"滤波后的历史数据":dbl[][])  [unwired: 2 in]
      }
    }
    n379 = node-c288() -> ()  [unwired: 1 in, 1 out]
  }
  n380 = while "While循环" {
    shift-right: [w512] -> _
    shift-left: enum16{"Init", "Event", "Exit"}."Init" -> [w513]
    stop <- w514 stop-if-true
    # "主框架"
    n381 = case shown="\"Event\"" w513 {
      tunnel: [FALSE FALSE TRUE] -> w514
      tunnel: [enum16{"Init", "Event", "Exit"}."Event" w538 enum16{"Init", "Event", "Exit"}."Exit"] -> w512
      frame "Init", Default {
        w517 = FALSE
        w520 = 0.0 ("TX")
        w528 = 0
        n382 = local read "WebBrowser"() -> (w516:refnum<k7>)
        n383 = invoke class="IWebBrowser2" method="Navigate"(reference=w516, "URL"="www.map.baidu.com") -> ()  [unwired: 6 in, 8 out]
        n384 = property on="波形图" class="WFGraph (严格)"("XScale.Maximum"=100, "XScale.Minimum"=0, "YScale.Maximum"=100, "YScale.Minimum"=-100) -> ()  [unwired: 2 in, 2 out]
        n385 = local write "FA数据接收（字符消息）"("Receive Area") -> ()
        n386 = local write "滤波系数调整"(3) -> ()
        n387 = local write "G值校准常量"(16600.0 ("RX")) -> ()
        n388 = local write "误码"(FALSE) -> ()
        n389 = local write "串口状态"(FALSE) -> ()
        n390 = local write "open"(FALSE) -> ()
        n391 = local write "发送区"("Send Area" ("发送区")) -> ()
        n392 = local write "TX"(0.0 ("TX")) -> ()
        n393 = local write "RX"(0.0 ("RX")) -> ()
        n394 = local write "计数器"(0) -> ()
        n395 = property on="波特率" class="Ring (严格)"("DisabledEnum"=w528) -> ()  [unwired: 2 in, 2 out]
        n396 = property on="VISA资源名称" class="VISAName"("DisabledEnum"=w528) -> ()  [unwired: 2 in, 2 out]
        n397 = local write "地图缩放"(17) -> ()
        n398 = property on="波形图" class="WFGraph (严格)"("Cursor.Cursor X"=w520, "Cursor.Cursor Y"=w520, "Cursor.Visible"=w517) -> ()  [unwired: 2 in, 2 out]
        n399 = property on="定位模式" class="Str"("Blinking"=w517) -> ()  [unwired: 2 in, 2 out]
        n400 = property on="档位" class="DigNum (严格)"("NumText.FontSize"=50) -> ()  [unwired: 2 in, 2 out]
      }
      frame "Event" {
        n401 = event shown="[3] 菜单选择(用户)" {
          selector: _ -> [_ _ _ _ _ _ _ _ _]
          dyn-events: _ -> [_ _ _ _ _ _ _ _ _]
          timeout: _ -> [_ _ _ _ _ _ _ _ _]
          tunnel: [enum16{"Init", "Event", "Exit"}."Event" enum16{"Init", "Event", "Exit"}."Event" enum16{"Init", "Event", "Exit"}."Event" enum16{"Init", "Event", "Exit"}."Event" enum16{"Init", "Event", "Exit"}."Event" enum16{"Init", "Event", "Exit"}."Event" enum16{"Init", "Event", "Exit"}."Event" enum16{"Init", "Event", "Exit"}."Event" enum16{"Init", "Event", "Exit"}."Event"] -> w538
          event "open": Value Change {
            # "目前有一个怀疑的BUG：\n由于是多while并列执行，\n多个while都有串口操作当\n虽然有if判断开关，再执行\n串口操作，但是在进入if后\n才触发了关闭串口事件，那\n么可能会导致串口已经关闭，\n但是仍然执行串口发送或者\n读取操作，可能这是导致关\n闭串口偶尔假死的原因。"
            n402 = event-data() -> ()  [unwired: 1 in, 5 out]
            n403 = disable-structure shown="启用" {
              disable-tunnel: ["VISA资源名称" _] -> w540
              frame Enabled {
              }
              frame Disabled {
                n404 = local read "端口号"() -> (w544:u16)
                n405 = case shown="5" w544 {
                  tunnel: [refnum<visa-resource-name> "ASRL1::INSTR" ("VISA resource name") refnum<visa-resource-name> "ASRL2::INSTR" ("VISA resource name") refnum<visa-resource-name> "ASRL3::INSTR" ("VISA resource name") refnum<visa-resource-name> "ASRL4::INSTR" ("VISA resource name") refnum<visa-resource-name> "ASRL5::INSTR" ("VISA resource name") refnum<visa-resource-name> "COM6" ("VISA resource name") refnum<visa-resource-name> "COM7" ("VISA resource name") refnum<visa-resource-name> "COM8" ("VISA resource name") refnum<visa-resource-name> "COM9" ("VISA resource name") refnum<visa-resource-name> "COM10" ("VISA resource name")] -> _
                  frame 0, Default {
                  }
                  frame 1 {
                  }
                  frame 2 {
                  }
                  frame 3 {
                  }
                  frame 4 {
                  }
                  frame 5 {
                  }
                  frame 6 {
                  }
                  frame 7 {
                  }
                  frame 8 {
                  }
                  frame 9 {
                  }
                }
              }
            }
            n406 = case shown="真" "open" {
              tunnel: w540 -> [w557 w563]
              frame False {
                w555 = 0
                n407 = local read "串口状态"() -> (w556:bool)
                n408 = case shown="真" w556 {
                  tunnel: w557 -> [_ w559]
                  frame False {
                  }
                  frame True {
                    w558 = FALSE
                    n409 = VISA Close(VISA resource name=w559) -> (error out=w560:errorcluster)  [unwired: 1 in]
                    n410 = local write "串口状态"(w558) -> ()
                    n411 = local write "计时开关"(w558) -> ()
                    n412 = call <vilib>:"Simple Error Handler.vi"("error in (no error)"=w560) -> ()  [unwired: 4 in, 5 out]
                  }
                }
                n413 = property on="波特率" class="Ring (严格)"("DisabledEnum"=w555) -> ()  [unwired: 2 in, 2 out]
                n414 = property on="VISA资源名称" class="VISAName"("DisabledEnum"=w555) -> ()  [unwired: 2 in, 2 out]
                n415 = property on="端口号" class="Ring (严格)"("DisabledEnum"=w555) -> ()  [unwired: 2 in, 2 out]
              }
              frame True {
                w561 = 2
                w565 = FALSE  # 无终止符
                w572 = u16 0  # 流控制
                w571 = u16 10  # 停止位
                w570 = u8 0  # 奇偶位
                w569 = u16 8  # 数据位
                n416 = case shown="0, 默认" "波特率" {
                  tunnel: [115200 9600] -> w568
                  frame 0, Default {
                  }
                  frame 1 {
                  }
                }
                n417 = call-poly "VISA Configure Serial Port"("VISA resource name"=w563, "Enable Termination\nChar (T)"=w565, "baud rate (9600)"=w568, "data bits (8)"=w569, "parity (0:none)"=w570, "stop bits (10: 1 bit)"=w571, "flow control (0:none)"=w572) -> ("error out"=w573:errorcluster)  [unwired: 7 in, 1 out]
                n418 = call <vilib>:"Simple Error Handler.vi"("type of dialog (OK msg:1)"=0, "error in (no error)"=w573) -> ("error?"=w566:bool)  [unwired: 3 in, 4 out]
                n419 = case shown="真" w566 {
                  tunnel: w563 -> [_ w575]
                  frame False {
                  }
                  frame True {
                    w574 = 0
                    n420 = One Button Dialog(message="串口不存在或已打开！") -> ()  [unwired: 1 in, 1 out]
                    n421 = local write "open"(FALSE) -> ()
                    n422 = property on="波特率" class="Ring (严格)"("DisabledEnum"=w574) -> ()  [unwired: 2 in, 2 out]
                    n423 = property on="VISA资源名称" class="VISAName"("DisabledEnum"=w574) -> ()  [unwired: 2 in, 2 out]
                    n424 = VISA Close(VISA resource name=w575) -> ()  [unwired: 1 in, 1 out]
                    n425 = property on="端口号" class="Ring (严格)"("DisabledEnum"=w574) -> ()  [unwired: 2 in, 2 out]
                  }
                }
                n426 = Not(x=w566) -> (.not. x?=w562:bool)
                "串口状态" <- w562
                n427 = local write "计时开关"(w562) -> ()
                n428 = property on="波特率" class="Ring (严格)"("DisabledEnum"=w561) -> ()  [unwired: 2 in, 2 out]
                n429 = property on="VISA资源名称" class="VISAName"("DisabledEnum"=w561) -> ()  [unwired: 2 in, 2 out]
                n430 = property on="端口号" class="Ring (严格)"("DisabledEnum"=w561) -> ()  [unwired: 2 in, 2 out]
              }
            }
          }
          event "send": Mouse Down {
            n431 = event-data() -> ()  [unwired: 1 in, 7 out]
            n432 = local read "串口状态"() -> (w581:bool)
            n433 = case shown="真" w581 {
              frame False {
              }
              frame True {
                n434 = disable-structure shown="启用" {
                  disable-tunnel: [w591 _] -> w582
                  frame Enabled {
                    n435 = local read "VISA资源名称"() -> (w591:refnum<visa-resource-name>)
                  }
                  frame Disabled {
                    n436 = local read "端口号"() -> (w592:u16)
                    n437 = case shown="5" w592 {
                      tunnel: [refnum<visa-resource-name> "ASRL1::INSTR" ("VISA resource name") refnum<visa-resource-name> "ASRL2::INSTR" ("VISA resource name") refnum<visa-resource-name> "ASRL3::INSTR" ("VISA resource name") refnum<visa-resource-name> "ASRL4::INSTR" ("VISA resource name") refnum<visa-resource-name> "ASRL5::INSTR" ("VISA resource name") refnum<visa-resource-name> "COM6" ("VISA resource name") refnum<visa-resource-name> "COM7" ("VISA resource name") refnum<visa-resource-name> "COM8" ("VISA resource name") refnum<visa-resource-name> "COM9" ("VISA resource name") refnum<visa-resource-name> "COM10" ("VISA resource name")] -> _
                      frame 0, Default {
                      }
                      frame 1 {
                      }
                      frame 2 {
                      }
                      frame 3 {
                      }
                      frame 4 {
                      }
                      frame 5 {
                      }
                      frame 6 {
                      }
                      frame 7 {
                      }
                      frame 8 {
                      }
                      frame 9 {
                      }
                    }
                  }
                }
                n438 = case shown="真" "换行" {
                  tunnel: [_ "\r"] -> w590
                  tunnel: [_ "\n"] -> w589
                  frame False {
                  }
                  frame True {
                  }
                }
                n439 = Concatenate Strings("发送区", w590, w589) -> (w586:string)
                n440 = local read "TX"() -> (w585:dbl)
                n441 = VISA Write(VISA resource name=w582, write buffer=w586) -> (return count=w583:u32)  [unwired: 1 in, 2 out]
                n442 = Add(x=w583, y=w585) -> (x+y=→"TX":dbl)
              }
            }
          }
          event "清除数据": Mouse Down {
            w611 = 0.0 ("RX")
            w605 = 0.0 ("RX")
            w610 = i16[][] []
            n443 = event-data() -> ()  [unwired: 1 in, 7 out]
            n444 = local write "轮速0"(w605) -> ()
            n445 = local write "水温"(w605) -> ()
            n446 = local write "纬度"(w605) -> ()
            n447 = local write "侧向加速度"(w605) -> ()
            n448 = local write "侧向角速度"(w605) -> ()
            n449 = local write "卫星数量"(w605) -> ()
            n450 = local write "档位"(w605) -> ()
            n451 = local write "地速"(w605) -> ()
            n452 = local write "电池电压"(w605) -> ()
            n453 = local write "海拔"(w605) -> ()
            n454 = local write "节流阀位置"(w605) -> ()
            n455 = local write "经度"(w605) -> ()
            n456 = local write "前向加速度"(w605) -> ()
            n457 = local write "前向角速度"(w605) -> ()
            n458 = local write "时间差"(w605) -> ()
            n459 = local write "转速"(w605) -> ()
            n460 = local write "纵向加速度"(w605) -> ()
            n461 = local write "纵向角速度"(w605) -> ()
            n462 = local write "时间差"(w605) -> ()
            n463 = Bundle("RX"=w611, "RX"=w611) -> (w612:cluster{"RX":dbl, "RX":dbl})  [unwired: 1 in]
            n464 = local write "侧向G值"(w612) -> ()
            n465 = local write "FA数据接收（字符消息）"("") -> ()
            n466 = property on="波形图" class="WFGraph (严格)"("XScale.Maximum"=100.0 ("RX"), "XScale.Minimum"=0.0 ("RX"), "YScale.Maximum"=100.0 ("RX"), "YScale.Minimum"=-100.0 ("RX")) -> ()  [unwired: 2 in, 2 out]
            n467 = local write "RX"(0.0 ("RX")) -> ()
            n468 = local write "TX"(0.0 ("RX")) -> ()
            n469 = local write "波形图"(w610) -> ()
            n470 = local write "滤波后的历史数据"(w610) -> ()
            n471 = local write "历史数据01"(w610) -> ()
            n472 = local write "历史数据02"(w610) -> ()
            n473 = local write "历史数据03"(w610) -> ()
            n474 = local write "历史数据04"(w610) -> ()
            n475 = local write "历史数据05"(w610) -> ()
            n476 = local write "历史数据F1"(w610) -> ()
            n477 = local write "历史数据F2"(w610) -> ()
            "存读的历史数据" <- w610
          }
          event Menu Selection (User) {
            n478 = event-data() -> ("ItemTag"=w617:string)  [unwired: 1 in, 5 out]
            n479 = case shown="\"协议\"" w617 {
              frame "假", Default {
              }
              frame "开发者信息" {
                n480 = One Button Dialog(message="青岛理工大学\nDRINOW\nEmail：yyh123@vip.qq.com\n2016.05\n" ("Message")) -> ()  [unwired: 1 in, 1 out]
              }
              frame "协议" {
                n481 = call <vilib>:"Application Directory.vi"() -> ("Application Directory"=w620:path)
                n482 = call <vilib>:"System Exec.vi"("wait until completion? (T)"=FALSE, "working directory"=w620, "command line"="cmd /c start 数据协议.xls") -> ("error out"=w622:errorcluster)  [unwired: 5 in, 3 out]
                n483 = call <vilib>:"Simple Error Handler.vi"("error in (no error)"=w622) -> ()  [unwired: 4 in, 5 out]
                n484 = One Button Dialog(message="功能帧02包含三轴加速度和三轴角速度\n功能帧04包含GPS相关数据\n功能帧05包含电压电流数据\n功能帧F1包含ECU相关数据\n功能帧F2包含ADC相关数据\n功能帧FA包含字符串显示数据" ("Message")) -> ()  [unwired: 1 in, 1 out]
              }
              frame "使用说明" {
                n485 = One Button Dialog(message="1.保存和读取按钮只能操作曲线数据，也只能复现曲线数据。\n\n2.在选择串口时，系统会自动搜寻可用串口，会造成暂时的卡顿，请稍候。\n\n3.关闭应用前，请先关闭串口，否则可能导致蓝屏事故！\n\n4.显示过多曲线会严重降低性能，导致丢失数据，请实时监测时只观看必要的曲线，建议不超过6条同时显示，未显示的数据仍会在后台记录，届时保存曲线即可！\n\n5.曲线数据是显示的原始数据，未加处理，比如电池电压数据显示1224是正常的，因为它是放大100倍后发送而来，它其实是指12.24V。但并不是所有数据都是放大100倍，有的只放大10倍。因此需注意甄别，保存曲线后会标明放大倍数。\n\n\nBUG反馈请联系青特车队电气组。" ("Message")) -> ()  [unwired: 1 in, 1 out]
              }
              frame "更新日志" {
                n486 = One Button Dialog(message="2016.5：完成初步版本。\n2016.6：修改了一些错误；增加了曲线保存数量；增加了滤波算法。\n2016.7：进行了一些优化；修改了一些错误；初步的测试；并增加了地图功能。\n2016.07.13：地图增加了滚轮缩放动作；增加了新的数据协议FA功能帧。\n2016.07.15：增加了GPS坐标到百度坐标的转换；进行了一些优化。\n" ("Message")) -> ()  [unwired: 1 in, 1 out]
              }
            }
          }
          event "WebBrowser": Mouse Wheel {
            n487 = event-data() -> ("Delta"=w629:i32)  [unwired: 1 in, 9 out]
            n488 = Greater Than 0?(x=w629) -> (x > 0?=w627:bool)
            n489 = case "条件结构" shown="真" w627 {
              frame False {
                # "缩小"
                n490 = local read "地图缩放"() -> (w633:u8)
                n491 = Decrement(x=w633) -> (x-1=w630:u8)
                n492 = Greater?(x=w630, y=0) -> (0:w631:bool)
                n493 = case shown="假" w631 {
                  tunnel: w630 -> [_ w635]
                  frame False {
                    n494 = local write "地图缩放"(1) -> ()
                  }
                  frame True {
                    n495 = local write "地图缩放"(w635) -> ()
                  }
                }
              }
              frame True {
                # "放大"
                n496 = local read "地图缩放"() -> (w639:u8)
                n497 = Increment(x=w639) -> (x+1=w638:u8)
                n498 = Greater?(x=w638, y=19) -> (0:w636:bool)
                n499 = case shown="真" w636 {
                  tunnel: w638 -> [w640 _]
                  frame False {
                    n500 = local write "地图缩放"(w640) -> ()
                  }
                  frame True {
                    n501 = local write "地图缩放"(19) -> ()
                  }
                }
              }
            }
          }
          event "显示游标": Value Change {
            n502 = event-data() -> ("NewVal"=w643:bool)  [unwired: 1 in, 5 out]
            n503 = property on="波形图" class="WFGraph (严格)"("Cursor.Visible"=w643) -> ()  [unwired: 2 in, 2 out]
          }
          event "保存按钮": Mouse Up {
            n504 = event-data() -> ()  [unwired: 1 in, 8 out]
            n505 = Insert Into Array(array=string[] ["侧向加速度*1", "前向加速度*1", "纵向加速度*1", "侧向角速度*1", "前向角速度*1", "纵向角速度*1", "海拔*0.1m", "地速*0.01km/h", "RPM*1", "节流阀位置*0.1%", "岐管压强*0.1kPa", "空气温度*0.1℃", "水温*0.1℃", "Lambda1*0.001La", "电池电压*0.01V", "轮速0*0.1km/h", "轮速1*0.1km/h", "轮速2*0.1km/h", "轮速3*0.1km/h", "滑移率*0.1km/h", "档位*0.1=Gear"], new element=string[] ["悬架行程左前*1", "悬架行程左后*1", "悬架行程右后*1", "悬架行程右前*1", "ADC1*1", "ADC2*1", "ADC3*1", "ADC4*1", "电流型ADC1*1", "电流型ADC2*1", "电流型ADC3*1", "", "", "", "", "", "", "", "", "", ""]) -> (w645:string[])  [unwired: 1 in]
            n506 = Two Button Dialog(message="保存的文件用Excel打开。", 1:"不！", 2:"知道了！") -> (T button?=w647:bool)
            n507 = case shown="真" w647 {
              tunnel: w645 -> [_ w660]
              frame False {
              }
              frame True {
                n508 = call "文件对话框"() -> ("selected path"=w653:path, "cancelled"=w661:bool, "error out"=w659:errorcluster)  [unwired: 12 in, 1 out]
                n509 = Path To String(path=w653) -> (string=w656:string)
                n510 = Not(x=w661) -> (.not. x?=w657:bool)
                n511 = Concatenate Strings(w656, ".csv") -> (w654:string)
                n512 = String To Path(string=w654) -> (path=w652:path)
                n513 = case shown="真" w657 {
                  tunnel: w660 -> [_ w663]
                  tunnel: w652 -> [_ w662]
                  frame False {
                  }
                  frame True {
                    n514 = call-poly <vilib>:"Write To Spreadsheet File.vi"("delimiter (\\t)"=",", "1D data"=w663, "file path (dialog if empty)"=w662) -> ("new file path (Not A Path if cancelled)"=w666:path)  [unwired: 5 in]
                    n515 = local read "存读的历史数据"() -> (w667:i16[][])
                    n516 = call-poly <vilib>:"Write To Spreadsheet File.vi"("delimiter (\\t)"=",", "append to file? (new file:F)"=TRUE, "2D data"=w667, "file path (dialog if empty)"=w666) -> ()  [unwired: 4 in, 1 out]
                  }
                }
                n517 = call <vilib>:"Clear Errors.vi"("error in (no error)"=w659, "specific error code to clear (0: all)"=0) -> ()  [unwired: 4 in, 2 out]
              }
            }
          }
          event "读取按钮": Mouse Up {
            n518 = event-data() -> ()  [unwired: 1 in, 8 out]
            n519 = call "文件对话框2"() -> ("selected path"=w671:path, "exists"=w669:bool, "error out"=w670:errorcluster)  [unwired: 12 in, 1 out]
            n520 = call <vilib>:"Clear Errors.vi"("error in (no error)"=w670) -> ()  [unwired: 5 in, 2 out]
            n521 = case shown="真" w669 {
              tunnel: w671 -> [_ w675]
              frame False {
              }
              frame True {
                n522 = call-poly <vilib>:"Read From Spreadsheet File.vi"("delimiter (\\t)"=",", "file path (dialog if empty)"=w675) -> ("all rows"=w677:i64[][])  [unwired: 5 in, 4 out]
                n523 = local write "存读的历史数据"(w677) -> ()
                n524 = local read "存读的历史数据"() -> (w674:i16[][])
                n525 = Transpose 2D Array(2D array=w674) -> (transposed array=w673:i16[][])
                n526 = local write "波形图"(w673) -> ()
              }
            }
          }
          event "计时开关": Mouse Up {
            n527 = event-data() -> ()  [unwired: 1 in, 8 out]
            n528 = local read "计时开关"() -> (w679:bool)
            n529 = case shown="真" w679 {
              frame False {
              }
              frame True {
                n530 = call <vilib>:"High Resolution Relative Seconds.vi"() -> ("relative seconds"=→"基准时间":dbl)
              }
            }
          }
        }
      }
      frame "Exit" {
      }
    }
  }
  n531 = disable-structure shown="禁用" {
    frame Disabled {
      n532 = call <vilib>:"OpenHandle.vi"() -> ("client handle out"=w684:T5)  [unwired: 14 in, 1 out]
      n533 = Concatenate Strings("&ak=EpTZXvrzwEOoKaMGuChYbBM0bEaye5gV", "&service_id=120422", "&latitude=35.957904", "&longitude=120.220495", "&coord_type=3", "&loc_time=1469064795", "&entity_name=racecar") -> (w688:string)
      n534 = call-poly <vilib>:"POST.vi"("client handle"=w684, "url"="http://api.map.baidu.com/trace/v2/track/addpoint", "buffer"=w688) -> ("body"=→"字符串 2":string)  [unwired: 9 in, 3 out]
    }
    frame Enabled {
    }
  }
  n535 = node-c288(w9) -> ()  [unwired: 1 out]
  n536 = node-c288(w3) -> ()  [unwired: 1 out]
  n537 = node-c288(w5) -> ()  [unwired: 1 out]
  n538 = node-c288(w7) -> ()  [unwired: 1 out]
  n539 = node-c288(w1) -> ()  [unwired: 1 out]
